vi "graph.vi"(5 "Open":bool, 6 "FrontN":T1 {"Power" format="%.2g"; "Voltage" format="%.2g"; "Current" format="%.2g"; "Regulator" format="%.2g"; "Extra sensor" format="%.2g"; "Cold plate" format="%.2g"; "Set point" format="%.2g"; "Main sensor" format="%.2g"}, 7 "TopS":T1 {"Power" format="%.2g"; "Voltage" format="%.2g"; "Current" format="%.2g"; "Regulator" format="%.2g"; "Extra sensor" format="%.2g"; "Cold plate" format="%.2g"; "Set point" format="%.2g"; "Main sensor" format="%.2g"}, 8 "FrontS":T1 {"Power" format="%.2g"; "Voltage" format="%.2g"; "Current" format="%.2g"; "Regulator" format="%.2g"; "Extra sensor" format="%.2g"; "Cold plate" format="%.2g"; "Set point" format="%.2g"; "Main sensor" format="%.2g"}, 9 "BottomN":T1 {"Power" format="%.2g"; "Voltage" format="%.2g"; "Current" format="%.2g"; "Regulator" format="%.2g"; "Extra sensor" format="%.2g"; "Cold plate" format="%.2g"; "Set point" format="%.2g"; "Main sensor" format="%.2g"}, 10 "BottomS":T1 {"Power" format="%.2g"; "Voltage" format="%.2g"; "Current" format="%.2g"; "Regulator" format="%.2g"; "Extra sensor" format="%.2g"; "Cold plate" format="%.2g"; "Set point" format="%.2g"; "Main sensor" format="%.2g"}, 11 "TopN":T1 {"Power" format="%.2g"; "Voltage" format="%.2g"; "Current" format="%.2g"; "Regulator" format="%.2g"; "Extra sensor" format="%.2g"; "Cold plate" format="%.2g"; "Set point" format="%.2g"; "Main sensor" format="%.2g"}) -> ()   [LabVIEW 2010]
uses:
  controler_custer.ctl
panel:
  out "Waveform Graph":waveform(dbl)[](graph)
  # "Temeprature"
  # "Temeprature"
  # "Temeprature"
  # "Temeprature"
  # "Temeprature"
  # "Temeprature"
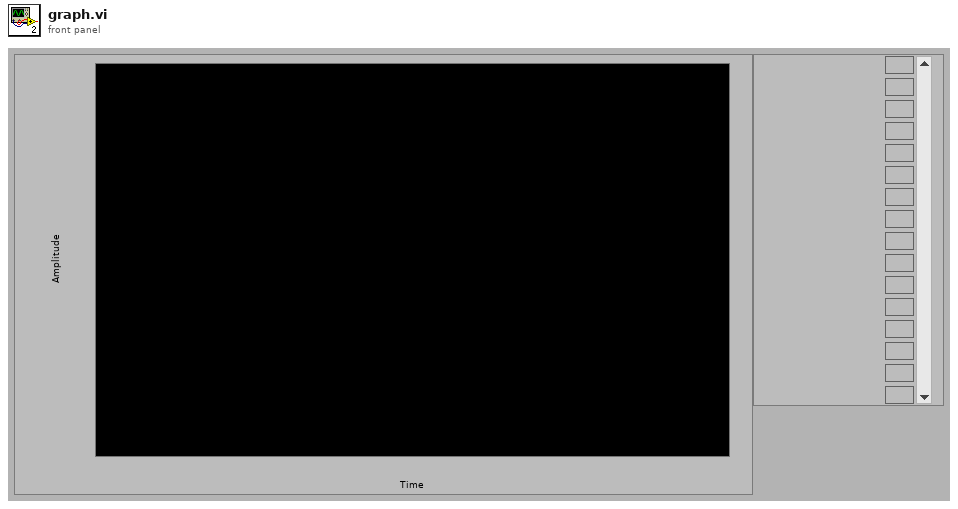
[diagram p1: front panel]
types:
  T1 = typedef "controler_custer.ctl" = cluster{"Set point":dbl, "Main sensor":dbl, "Cold plate":dbl, "Extra sensor":dbl, "Regulator":dbl, "Voltage":dbl, "Current":dbl, "Power":dbl}
  T2 = enum32{"Invalid", "Standard", "Closed", "Hidden", "Minimized", "Maximized"}
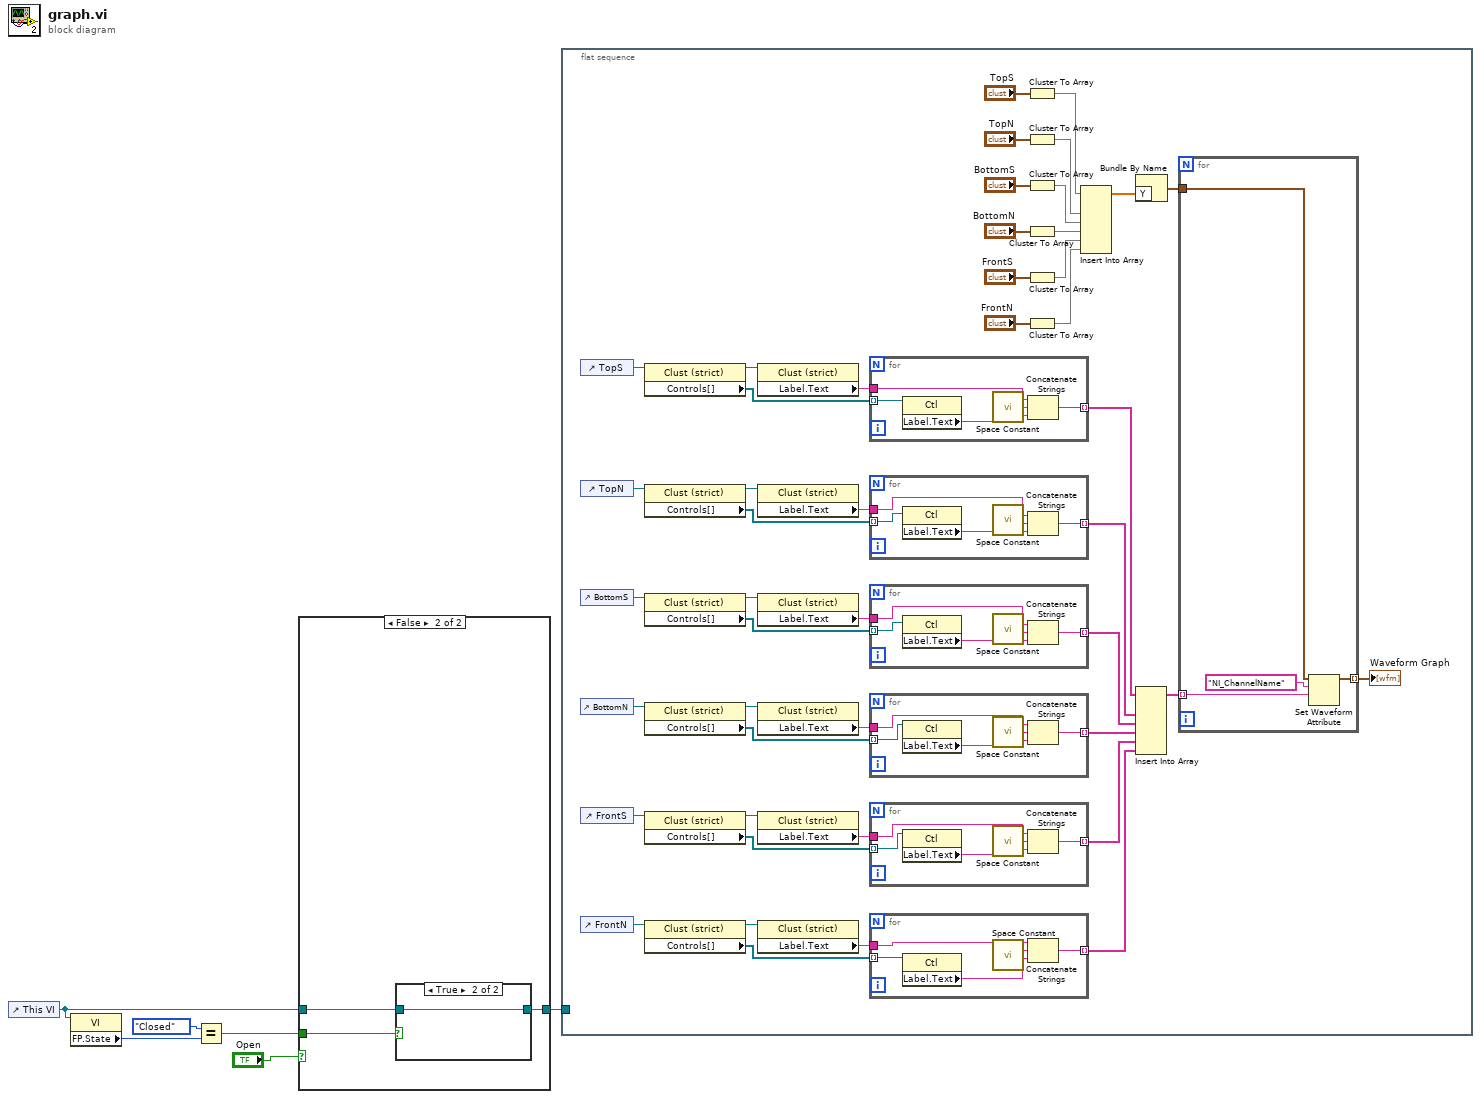
[diagram p0: block diagram]
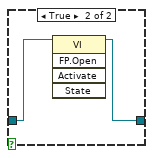
[diagram p3: hidden frame]
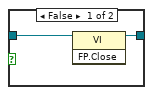
[diagram p4: hidden frame]
diagram:
  n1 = control-ref of="This VI"() -> (w5:refnum<vi>)
  n2 = property class="VI"(reference=w5) -> ("FP.State"=w4:T2)  [unwired: 1 in, 2 out]
  n3 = Equal?(x=T2."Closed", y=w4) -> (x = y?=w2:bool)
  n4 = case shown="False" "Open" {
    tunnel: w5 -> [w9 w14]
    tunnel: [w8 w13] -> w6
    tunnel: w2 -> [w7 w15]
    frame True {
      n5 = case shown="False" w7 {
        tunnel: w9 -> [w10 w12]
        tunnel: [w10 w11] -> w8
        frame False {
        }
        frame True {
          n6 = invoke class="VI" method="FP.Open"(reference=w12) -> (reference out=w11:refnum<vi>)  [unwired: 4 in, 4 out]
        }
      }
    }
    frame False {
      n7 = case shown="True" w15 {
        tunnel: w14 -> [w17 w18]
        tunnel: [w16 w18] -> w13
        frame False {
          n8 = invoke class="VI" method="FP.Close"(reference=w17) -> (reference out=w16:refnum<vi>)  [unwired: 2 in, 2 out]
        }
        frame True {
        }
      }
    }
  }
  n9 = flat-sequence {
    tunnel: w6 -> [_]
    frame #0 {
      n10 = control-ref of="TopS"() -> (w49:refnum<vi>)
      n11 = control-ref of="TopN"() -> (w48:refnum<vi>)
      n12 = control-ref of="BottomS"() -> (w47:refnum<vi>)
      n13 = control-ref of="BottomN"() -> (w44:refnum<vi>)
      n14 = control-ref of="FrontS"() -> (w45:refnum<vi>)
      n15 = control-ref of="FrontN"() -> (w46:refnum<vi>)
      n16 = property class="Clust (strict)"(reference=w49) -> (reference out=w43:refnum<vi>, "Controls[]"=w42:refnum<vi>[])  [unwired: 1 in, 1 out]
      n17 = property class="Clust (strict)"(reference=w48) -> (reference out=w39:refnum<vi>, "Controls[]"=w32:refnum<vi>[])  [unwired: 1 in, 1 out]
      n18 = property class="Clust (strict)"(reference=w47) -> (reference out=w38:refnum<vi>, "Controls[]"=w21:refnum<vi>[])  [unwired: 1 in, 1 out]
      n19 = property class="Clust (strict)"(reference=w44) -> (reference out=w37:refnum<vi>, "Controls[]"=w20:refnum<vi>[])  [unwired: 1 in, 1 out]
      n20 = property class="Clust (strict)"(reference=w45) -> (reference out=w36:refnum<vi>, "Controls[]"=w19:refnum<vi>[])  [unwired: 1 in, 1 out]
      n21 = property class="Clust (strict)"(reference=w46) -> (reference out=w35:refnum<vi>, "Controls[]"=w25:refnum<vi>[])  [unwired: 1 in, 1 out]
      n22 = property class="Clust (strict)"(reference=w43) -> ("Label.Text"=w41:string)  [unwired: 1 in, 2 out]
      n23 = property class="Clust (strict)"(reference=w39) -> ("Label.Text"=w33:string)  [unwired: 1 in, 2 out]
      n24 = property class="Clust (strict)"(reference=w38) -> ("Label.Text"=w22:string)  [unwired: 1 in, 2 out]
      n25 = property class="Clust (strict)"(reference=w37) -> ("Label.Text"=w23:string)  [unwired: 1 in, 2 out]
      n26 = property class="Clust (strict)"(reference=w36) -> ("Label.Text"=w24:string)  [unwired: 1 in, 2 out]
      n27 = property class="Clust (strict)"(reference=w35) -> ("Label.Text"=w26:string)  [unwired: 1 in, 2 out]
      n28 = for {
        tunnel: w42 -> [w94] mode=indexing
        tunnel: w41 -> [w91]
        tunnel: [w92] -> w40 mode=indexing
        n29 = property class="Ctl"(reference=w94) -> ("Label.Text"=w93:string)  [unwired: 1 in, 2 out]
        n30 = call <vilib>:"Space Constant.vi"() -> ("String"=w90:string)
        n31 = Concatenate Strings(w91, w90, w93) -> (w92:string)
      }
      n32 = for {
        tunnel: w32 -> [w89] mode=indexing
        tunnel: w33 -> [w86]
        tunnel: [w87] -> w31 mode=indexing
        n33 = property class="Ctl"(reference=w89) -> ("Label.Text"=w88:string)  [unwired: 1 in, 2 out]
        n34 = call <vilib>:"Space Constant.vi"() -> ("String"=w85:string)
        n35 = Concatenate Strings(w86, w85, w88) -> (w87:string)
      }
      n36 = for {
        tunnel: w21 -> [w84] mode=indexing
        tunnel: w22 -> [w81]
        tunnel: [w82] -> w30 mode=indexing
        n37 = property class="Ctl"(reference=w84) -> ("Label.Text"=w83:string)  [unwired: 1 in, 2 out]
        n38 = call <vilib>:"Space Constant.vi"() -> ("String"=w80:string)
        n39 = Concatenate Strings(w81, w80, w83) -> (w82:string)
      }
      n40 = for {
        tunnel: w20 -> [w79] mode=indexing
        tunnel: w23 -> [w76]
        tunnel: [w77] -> w29 mode=indexing
        n41 = property class="Ctl"(reference=w79) -> ("Label.Text"=w78:string)  [unwired: 1 in, 2 out]
        n42 = call <vilib>:"Space Constant.vi"() -> ("String"=w75:string)
        n43 = Concatenate Strings(w76, w75, w78) -> (w77:string)
      }
      n44 = for {
        tunnel: w24 -> [w72]
        tunnel: [w73] -> w28 mode=indexing
        tunnel: w19 -> [w70] mode=indexing
        n45 = property class="Ctl"(reference=w70) -> ("Label.Text"=w74:string)  [unwired: 1 in, 2 out]
        n46 = call <vilib>:"Space Constant.vi"() -> ("String"=w71:string)
        n47 = Concatenate Strings(w72, w71, w74) -> (w73:string)
      }
      n48 = for {
        tunnel: w25 -> [w69] mode=indexing
        tunnel: w26 -> [w66]
        tunnel: [w67] -> w27 mode=indexing
        n49 = property class="Ctl"(reference=w69) -> ("Label.Text"=w68:string)  [unwired: 1 in, 2 out]
        n50 = call <vilib>:"Space Constant.vi"() -> ("String"=w65:string)
        n51 = Concatenate Strings(w66, w65, w68) -> (w67:string)
      }
      n52 = Cluster To Array(cluster="TopS") -> (array=w62:dbl[])
      n53 = Cluster To Array(cluster="TopN") -> (array=w61:dbl[])
      n54 = Cluster To Array(cluster="BottomS") -> (array=w60:dbl[])
      n55 = Cluster To Array(cluster="BottomN") -> (array=w59:dbl[])
      n56 = Cluster To Array(cluster="FrontS") -> (array=w58:dbl[])
      n57 = Cluster To Array(cluster="FrontN") -> (array=w57:dbl[])
      n58 = Insert Into Array(array=w62, new element #1=w61, new element #2=w60, new element #3=w59, new element #4=w58, new element #5=w57) -> (w56:dbl[])  [unwired: 1 in]
      n59 = Bundle By Name("Y"=w56) -> (w63:waveform(dbl))  [unwired: 1 in]
      n60 = Insert Into Array(array=w40, new element #1=w31, new element #2=w30, new element #3=w29, new element #4=w28, new element #5=w27) -> (w34:string[])  [unwired: 1 in]
      n61 = for {
        tunnel: w63 -> [w98]
        tunnel: [w96] -> w64 mode=indexing
        tunnel: w34 -> [w95] mode=indexing
        n62 = Set Waveform Attribute(5:w95, 6:"NI_ChannelName" ("name"), 7:w98) -> (3:w96:waveform(dbl))  [unwired: 1 in, 2 out]
      }
      "Waveform Graph" <- w64
    }
  }
